vi "EMB Main Window .vi"() -> ()   [LabVIEW 2019]
uses:
  Servo Parameters.ctl
panel:
  out "NextState":T1(ring)
  out "Tab Control":T2(tab)
  in  "Servo Parameters":T3
  in  "Calibrate 2":bool
  out "Servo Current Force":dbl
  out "Servo Current Position":dbl
  in  "Exit":bool
  out "Current State":string
  in  "Login":bool
  in  "Reset":bool
  in  "Stop":bool
  in  "Start":bool
  # "EMB Force Calibrator Prototype\n\nElectrical drawing:  \nMechanical drawing:"
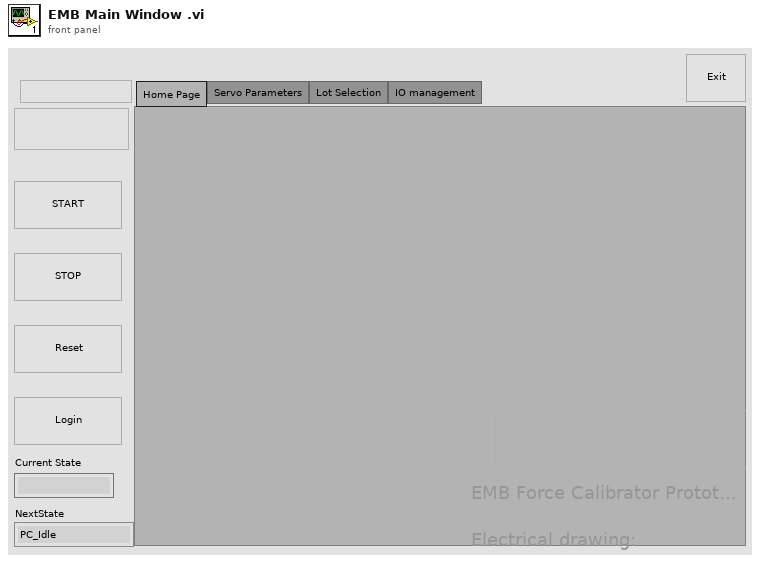
[diagram p1: front panel]
types:
  T1 = enum16{"PC_Idle", "Part_Load", "Part_Presence_Check", "Door_Closed", "LoadCellCalibration", "ServoMoveToApproachPosition", "ServoMoveToTargetPosition", "ServoMoveToHomePosition", "Doors_Open"}
  T2 = enum32{"Home Page", "Servo Parameters", "Lot Selection", "IO management"}
  T3 = typedef "Servo Parameters.ctl" = cluster{"Approch Servo Position":dbl, "Approch Speed":dbl, "Approch Acceleration":dbl, "Approch Deacceleration":dbl, "Target Servo Position ":dbl, "Target Speed ":dbl, "Target Acceleration ":dbl, "Target Deacceleration":dbl, "Target Force":dbl}
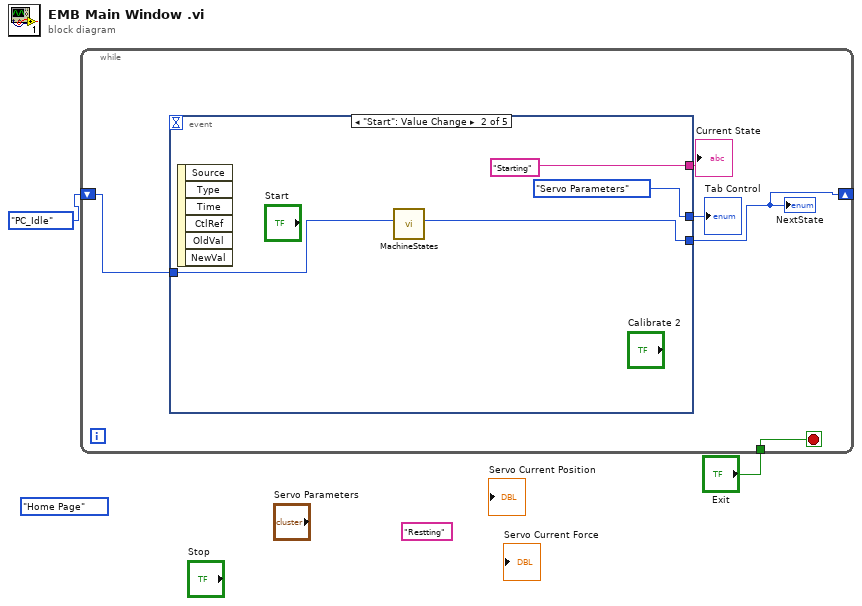
[diagram p0: block diagram]
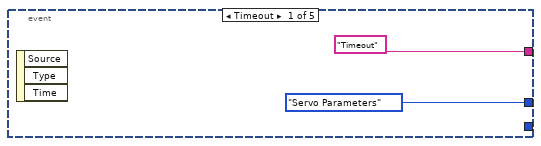
[diagram p2: hidden frame]
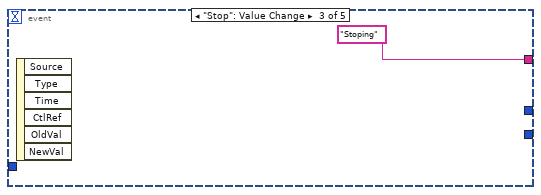
[diagram p3: hidden frame]
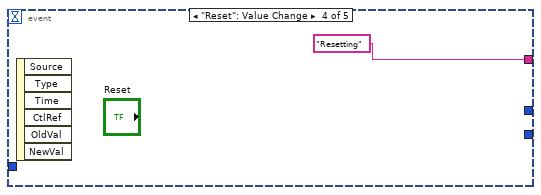
[diagram p4: hidden frame]
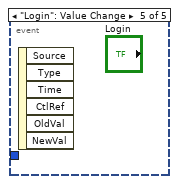
[diagram p5: hidden frame]
diagram:
  (unwired) T2."Home Page" ("Tab Control")
  (unwired) "Restting" ("String 2")
  n1 = while {
    tunnel: "Exit" -> [w6]
    shift-right: [w3] -> _
    shift-left: T1."PC_Idle" ("NextState") -> [w4]
    stop <- w6 stop-if-true
    n2 = event shown="[1] \"Start\": Value Change" {
      selector: _ -> [_ _ _ _ _]
      dyn-events: _ -> [_ _ _ _ _]
      timeout: _ -> [_ _ _ _ _]
      tunnel: ["Timeout" ("String 2") "Starting" ("String 2") "Stoping" ("String 2") "Resetting" ("String 2") _] -> w7
      tunnel: [T2."Servo Parameters" ("Tab Control") T2."Servo Parameters" ("Tab Control") _ _ _] -> w5
      tunnel: w4 -> [_ w11 _ _ _]
      tunnel: [_ w10 _ _ _] -> w3
      event Timeout {
        n3 = event-data() -> ()  [unwired: 1 in, 3 out]
      }
      event "Start": Value Change {
        n4 = event-data() -> ()  [unwired: 1 in, 6 out]
        n5 = call "MachineStates.vi"("MachineStates"=w11) -> ("NextStep"=w10:T1)  [unwired: 9 in, 1 out]
      }
      event "Stop": Value Change {
        n6 = event-data() -> ()  [unwired: 1 in, 6 out]
      }
      event "Reset": Value Change {
        n7 = event-data() -> ()  [unwired: 1 in, 6 out]
      }
      event "Login": Value Change {
        n8 = event-data() -> ()  [unwired: 1 in, 6 out]
      }
    }
    "Current State" <- w7
    "Tab Control" <- w5
    "NextState" <- w3
  }
